vi "stageOpen.vi"() -> (0 "stageError":errorcluster, 1 "stageIDs":cluster{"opaque pointer":u64, "id":i32})   [LabVIEW 2017]
uses:
  globalDevices.vi
  Stage/ximcLVx64/libximc.lvlib
panel:
  out "status out":T1
  in  "error in (no error)":errorcluster
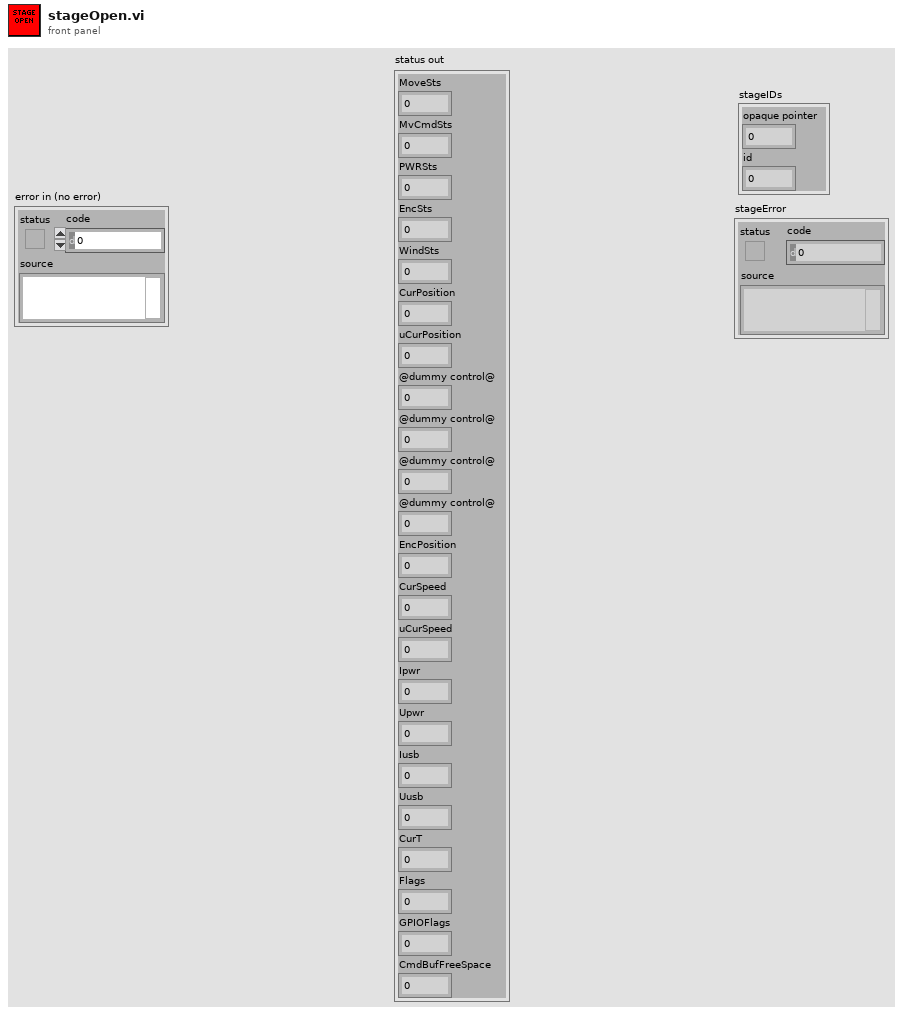
[diagram p1: front panel]
types:
  T1 = cluster{"MoveSts":u32, "MvCmdSts":u32, "PWRSts":u32, "EncSts":u32, "WindSts":u32, "CurPosition":i32, "uCurPosition":i32, "@dummy control@":i8, "@dummy control@":i8, "@dummy control@":i8, "@dummy control@":i8, "EncPosition":i64, "CurSpeed":i32, "uCurSpeed":i32, "Ipwr":i32, "Upwr":i32, "Iusb":i32, "Uusb":i32, "CurT":i32, "Flags":u32, "GPIOFlags":u32, "CmdBufFreeSpace":u32}
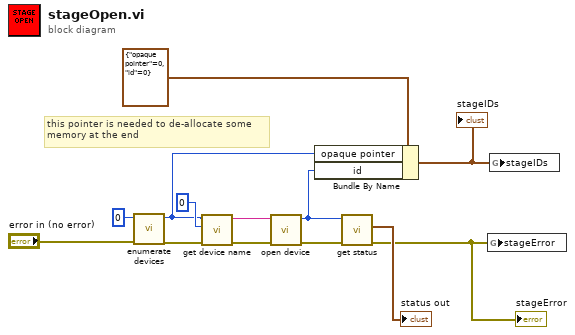
[diagram p0: block diagram]
diagram:
  # "this pointer is needed to de-allocate some\nmemory at the end"
  n1 = call "enumerate devices.vi"("error in (no error)"="error in (no error)", "enumerate_flags"=0) -> ("error out"=w6:errorcluster, "function return"=w7:u64)  [unwired: 8 in]
  n2 = call "get device name.vi"("error in (no error)"=w6, "device_index"=0, "device_enumeration"=w7) -> ("error out"=w10:errorcluster, "function return"=w11:string)  [unwired: 7 in]
  n3 = call "open device.vi"("error in (no error)"=w10, "name"=w11) -> ("error out"=w4:errorcluster, "function return"=w5:i32)  [unwired: 8 in]
  n4 = Bundle By Name(cluster=cluster{"opaque pointer":u64, "id":i32} {"opaque pointer"=0, "id"=0}, "opaque pointer"=w7, "id"=w5) -> (w2:cluster{"opaque pointer":u64, "id":i32})
  "stageIDs" <- w2
  n5 = call "get status.vi"("error in (no error)"=w4, "id"=w5) -> ("error out"=w1:errorcluster, "status out"=→"status out":T1)  [unwired: 7 in, 1 out]
  "stageError" <- w1
  n6 = global write "globalDevices.vi" "stageError"(w1) -> ()
  n7 = global write "globalDevices.vi" "stageIDs"(w2) -> ()
